vi "measure_j-v_keithley-2450.vi"(0 "User Name":string, 1 "Cell details cluster":T2={"Cell Position"=16, "Cell Label"="", "Pixel to measure"=0, "Area (cm^2)"=0.126, "Variable"="", "Variable value"="", "Scan settings in queue"=0, "Light or dark"="", "Measurement type"=""} {"Pixel to measure" items=["All", "1", "2", "3", "4", "5", "6", "7", "8"]}, 3 "Date array":string[](array[string]), 5 "Experiment Title":string, 12 "Scan settings":T1={"J-V scan"=TRUE, "Start voltage (V)"=0.0, "End voltage (V)"=0.0, "Step voltage (V)"=1.4, "Scan both directions"=TRUE, "Inverted device structure"=FALSE, "Settling delay (ms)"=10.0, "Measurement speed"=0, "Scan rate (V/s)"=0.0, "Stabilisation time (s)"=0.0, "Stabilisation mode"=0, "Stabilisation value (V or A) "=1.0, "Illumination"=0, "Stabilisation in the dark?"=FALSE, "Repeat light scans"=FALSE, "No. of repeat scans"=0.0, "Only repeat for best pixel"=1, "J-t scan"=FALSE, "J-t best pixel only"=7, "J-t start voltage (V)"=0.0, "J-t end voltage (V)"=1.4, "J-t step voltage (V)"=0.01, "Step time (s)"=0.7, "J-t scan both directions"=TRUE, "J-t inverted device structure"=FALSE, "J-t settling delay (ms)"=0.0, "J-t measurement speed"=0, "J-t illumination"=2, "Max. power stabilisation"=FALSE, "Max power best pixel only"=1, "Max. power point tracker"=FALSE, "Vmp from J-V scan"=FALSE, "Max P stab. Specific voltage"=FALSE, "Vmp (V)"=1.0, "Stabilisation time step (s)"=1.0, "Total stabilisation time (s)"=100.0} {"J-t settling delay (ms)" min=10.0; "J-t illumination" items=["Light only", "Dark only", "Light then dark", "Dark then light"]; "Measurement speed" items=["Fast", "Normal", "High accuracy"]; "Illumination" items=["Light only", "Dark only", "Light then dark", "Dark then light"]; "Only repeat for best pixel" items=["only for best pixel", "for best 2 pixels", "for best 3 pixels", "for best 4 pixels", "for best 5 pixels", "for best 6 pixels", "for best 7 pixels", "for all pixels"]; "No. of repeat scans" min=1.0 step=1.0; "Max power best pixel only" items=["only the best pixel", "the best 2 pixels", "the best 3 pixels", "the best 4 pixels", "the best 5 pixels", "the best 6 pixels", "the best 7 pixels", "all pixels"]; "J-t best pixel only" items=["only the best pixel", "the best 2 pixels", "the best 3 pixels", "the best 4 pixels", "the best 5 pixels", "the best 6 pixels", "the best 7 pixels", "all pixels"]; "J-t measurement speed" items=["Fast", "Normal", "High Accuracy"]; "Stabilisation mode" items=["V", "I"]; "Settling delay (ms)" min=10.0}, 13 "VISA resource name":refnum<visa-resource-name>="GPIB1::24::INSTR", 14 "Skip pixel?":bool) -> (4 "JV Curve":cluster{"Y":dbl[], "Y":dbl[]}[](graph), 6 "File path for master log":path, 15 "Log Table":string[][](table))   [LabVIEW 2016]
uses:
  <instrlib>/Keithley 2450/Keithley 2450.lvlib
  TypeDefs/scan_settings.ctl
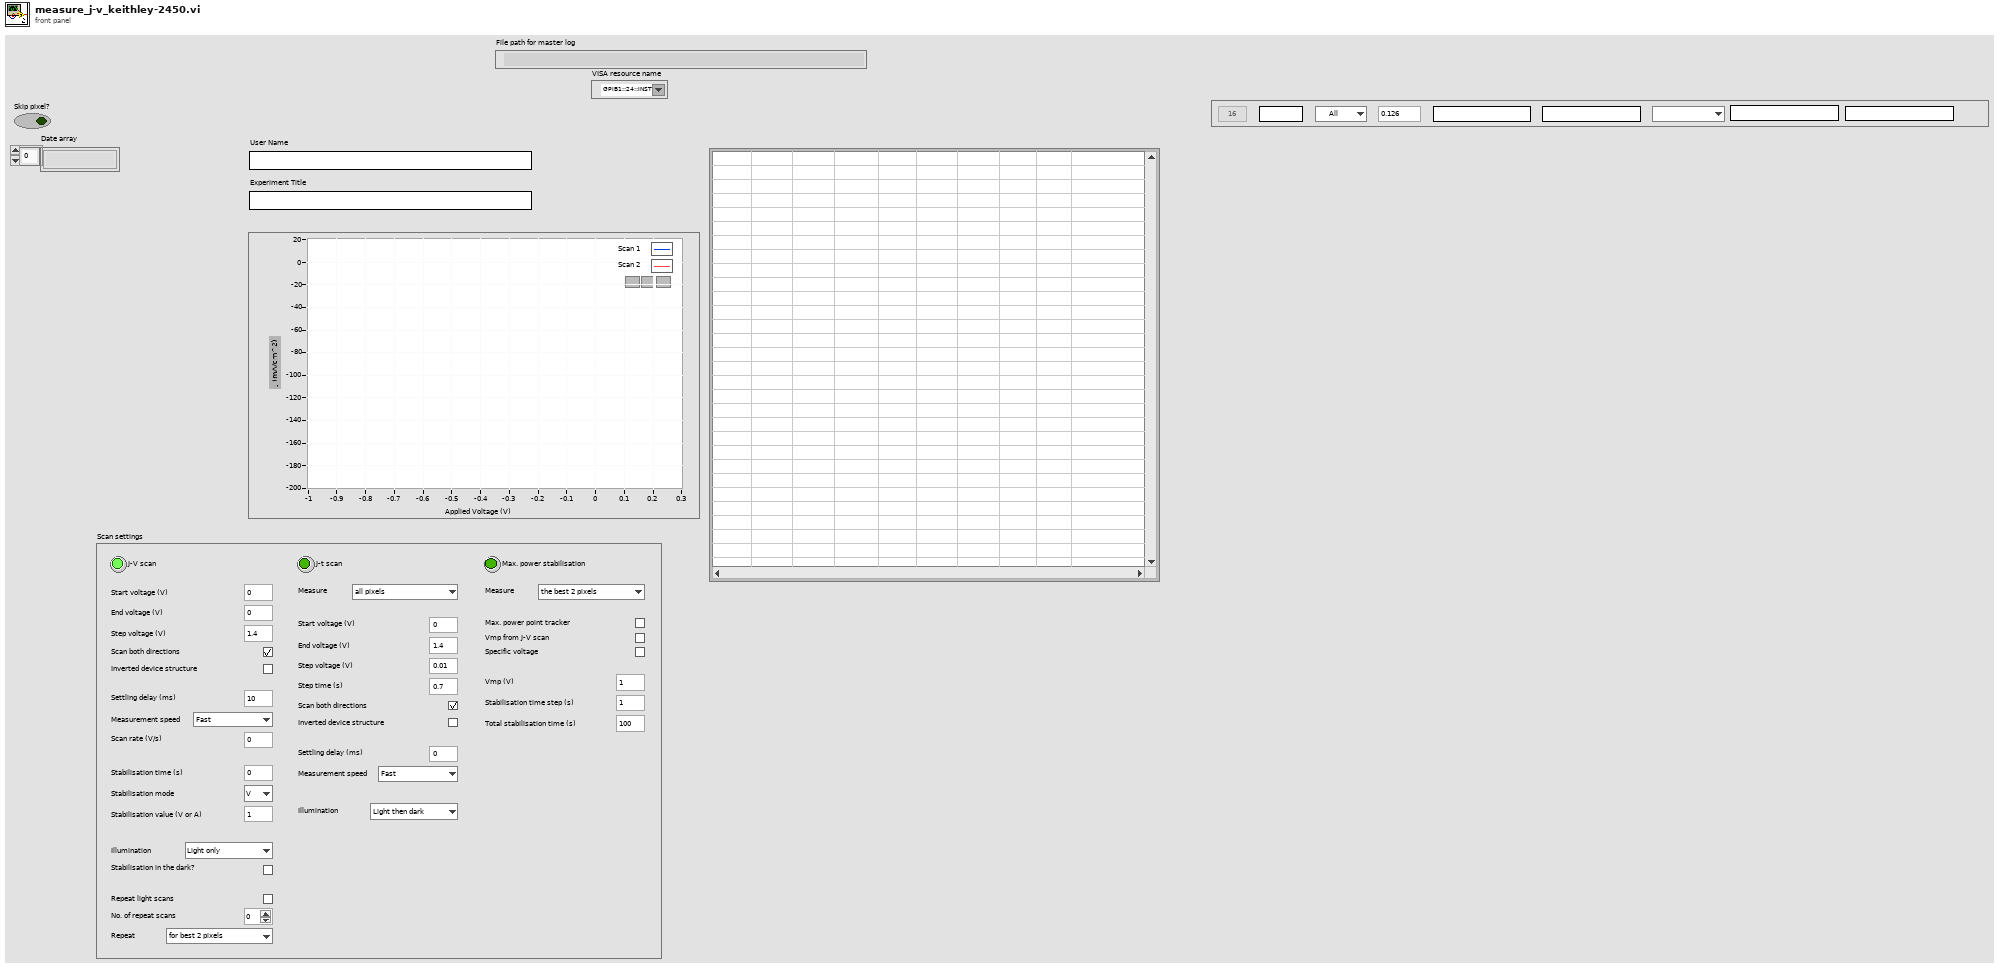
[diagram p1: front panel]
types:
  T1 = typedef "scan_settings.ctl" = cluster{"J-V scan":bool, "Start voltage (V)":dbl, "End voltage (V)":dbl, "Step voltage (V)":dbl, "Scan both directions":bool, "Inverted device structure":bool, "Settling delay (ms)":dbl, "Measurement speed":u8, "Scan rate (V/s)":dbl, "Stabilisation time (s)":dbl, "Stabilisation mode":u16, "Stabilisation value (V or A) ":dbl, "Illumination":u16, "Stabilisation in the dark?":bool, "Repeat light scans":bool, "No. of repeat scans":dbl, "Only repeat for best pixel":u16, "J-t scan":bool, "J-t best pixel only":u16, "J-t start voltage (V)":dbl, "J-t end voltage (V)":dbl, "J-t step voltage (V)":dbl, "Step time (s)":dbl, "J-t scan both directions":bool, "J-t inverted device structure":bool, "J-t settling delay (ms)":dbl, "J-t measurement speed":u16, "J-t illumination":u16, "Max. power stabilisation":bool, "Max power best pixel only":u16, "Max. power point tracker":bool, "Vmp from J-V scan":bool, "Max P stab. Specific voltage":bool, "Vmp (V)":dbl, "Stabilisation time step (s)":dbl, "Total stabilisation time (s)":dbl}
  T2 = cluster{"Cell Position":i32, "Cell Label":string, "Pixel to measure":u16, "Area (cm^2)":dbl, "Variable":string, "Variable value":string, "Scan settings in queue":u16, "Light or dark":string, "Measurement type":string}
  T3 = typedef "imagedata.ctl" = cluster{"image type":i32, "image depth":i32, "image":u8[], "mask":u8[], "colors":u32[], "Rectangle":cluster{"left":i16, "top":i16, "right":i16, "bottom":i16}}
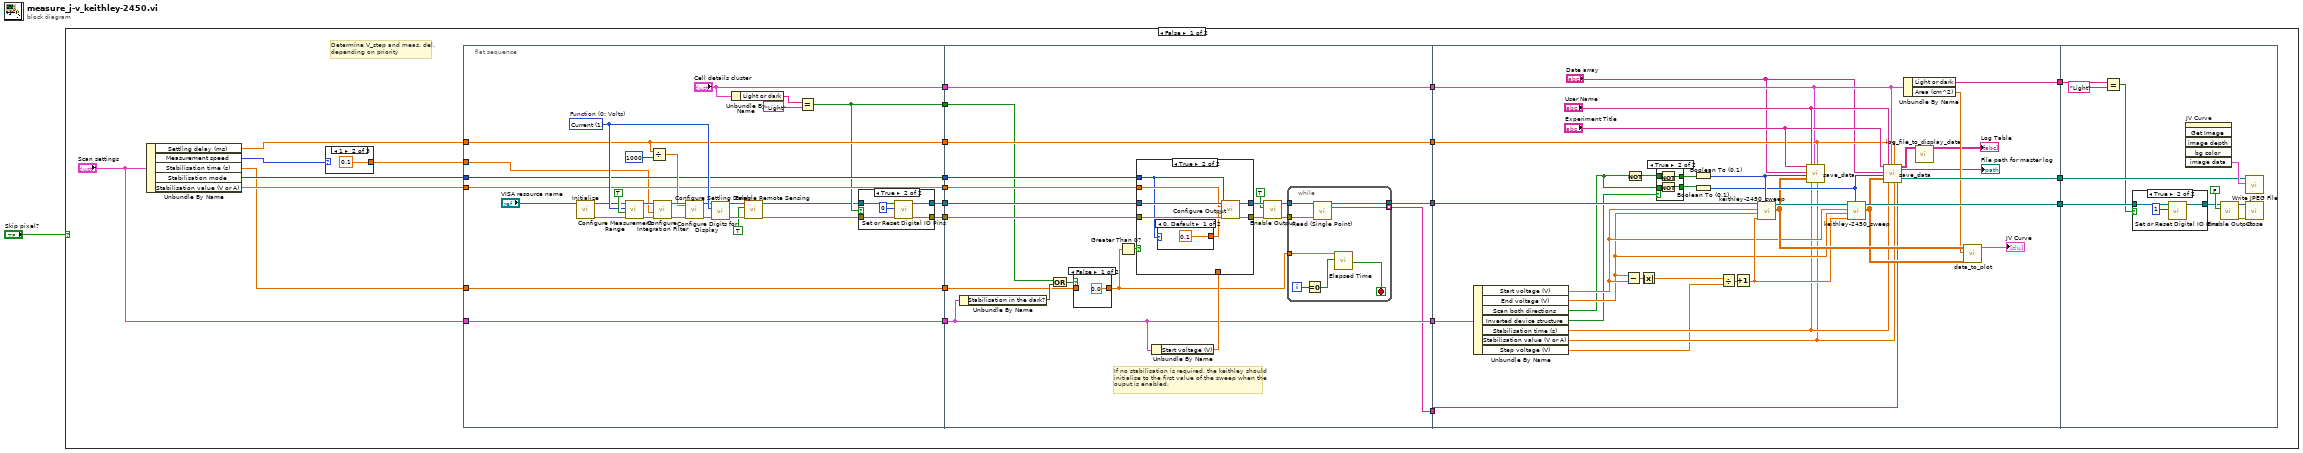
[diagram p0: block diagram]
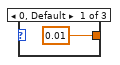
[diagram p2: hidden frame]
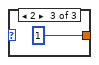
[diagram p3: hidden frame]
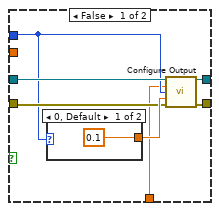
[diagram p6: hidden frame]
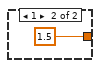
[diagram p7: hidden frame]
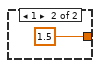
[diagram p8: hidden frame]
diagram:
  n1 = case shown="False" "Skip pixel?" {
    frame False {
      # "Determine V_step and meas. del.\ndepending on priority"
      n2 = Unbundle By Name("Scan settings") -> ("Settling delay (ms)"=w2:dbl, "Measurement speed"=w3:u8, "Stabilisation time (s)"=w5:dbl, "Stabilisation mode"=w7:u16, "Stabilisation value (V or A)"=w8:dbl)
      n3 = case shown="1" w3 {
        tunnel: [0.01 0.1 1] -> w4
        frame 0, Default {
        }
        frame 1 {
        }
        frame 2 {
        }
      }
      n4 = flat-sequence {
        tunnel: [w42] -> w25
        tunnel: [w35] -> w24
        tunnel: [w36] -> w23
        tunnel: w8 -> [w42]
        tunnel: [w41] -> w22
        tunnel: w7 -> [w41]
        tunnel: [w40] -> w21
        tunnel: w5 -> [w40]
        tunnel: w2 -> [w39]
        tunnel: [w39] -> w20
        tunnel: [w38] -> w19
        tunnel: "Scan settings" -> [w38]
        tunnel: ["Cell details cluster"] -> w18
        tunnel: [w32] -> w17
        tunnel: w4 -> [w31]
        tunnel: w25 -> [w78]
        tunnel: w24 -> [w83]
        tunnel: w23 -> [w84]
        tunnel: [w79] -> w16
        tunnel: [w66] -> w15
        tunnel: w22 -> [w75]
        tunnel: w21 -> [w67]
        tunnel: [w77] -> w14
        tunnel: w20 -> [w77]
        tunnel: [w72] -> w13
        tunnel: w19 -> [w72]
        tunnel: [w76] -> w12
        tunnel: w18 -> [w76]
        tunnel: w17 -> [w70]
        tunnel: [w142] -> w11
        tunnel: [w135] -> w10
        tunnel: w16 -> [w149]
        tunnel: w15 -> [w134]
        tunnel: w14 -> [w131]
        tunnel: w13 -> [w130]
        tunnel: w12 -> [w124]
        tunnel: [w123] -> w9
        tunnel: w11 -> [w160]
        tunnel: w10 -> [w161]
        tunnel: w9 -> [w156]
        frame #0 {
          w54 = u16 1 items=["Volts", "Current", "Resistance"]  # Function (0: Volts)
          n5 = call <instrlib>:"Initialize.vi"("VISA resource name"="VISA resource name") -> ("error out"=w44:errorcluster, "VISA resource name out"=w45:refnum<visa-resource-name>)  [unwired: 9 in]
          n6 = call <instrlib>:"Configure Measurement Range.vi"("error in (no error)"=w44, "Enable Auto Range (T:Enable)"=TRUE, "Function (0: Volts)"=w54, "VISA resource name"=w45) -> ("error out"=w47:errorcluster, "VISA resource name out"=w46:refnum<visa-resource-name>)  [unwired: 6 in]
          n7 = Divide(x=w39, y=1000) -> (x/y=w53:dbl)
          n8 = call <instrlib>:"Configure Integration Filter.vi"("error in (no error)"=w47, "Measurement Speed (1 PLC)"=w31, "VISA resource name"=w46) -> ("error out"=w56:errorcluster, "VISA resource name out"=w55:refnum<visa-resource-name>)  [unwired: 7 in]
          n9 = call <instrlib>:"Configure Settling Delay.vi"("Function (0: Volts)"=w53, "error in (no error)"=w56, "VISA resource name"=w55) -> ("error out"=w51:errorcluster, "VISA resource name out"=w50:refnum<visa-resource-name>)  [unwired: 7 in]
          n10 = call <instrlib>:"Configure Digits for Display.vi"("error in (no error)"=w51, "Function (0: Volts)"=w54, "VISA resource name"=w50) -> ("error out"=w49:errorcluster, "VISA resource name out"=w48:refnum<visa-resource-name>)  [unwired: 7 in]
          n11 = Unbundle By Name("Cell details cluster") -> ("Light or dark"=w34:string)
          n12 = call <instrlib>:"Enable Remote Sensing.vi"("error in (no error)"=w49, "Enable Remote Sensing (T: Enable)"=TRUE ("Enable Output (T: Enable)"), "VISA resource name"=w48) -> ("error out"=w29:errorcluster, "VISA resource name out"=w30:refnum<visa-resource-name>)  [unwired: 7 in]
          n13 = Equal?(x=w34, y="Light") -> (x = y?=w32:bool)
          n14 = case shown="True" w32 {
            tunnel: w30 -> [w60 w64]
            tunnel: w29 -> [w59 w63]
            tunnel: [w60 w62] -> w36
            tunnel: [w59 w61] -> w35
            frame False {
            }
            frame True {
              n15 = call <instrlib>:"Set or Reset Digital IO Pins.vi"("error in (no error)"=w63, "Digital IO Line (1)"=0, "VISA resource name"=w64) -> ("error out"=w61:errorcluster, "VISA resource name out"=w62:refnum<visa-resource-name>)  [unwired: 7 in]
            }
          }
        }
        frame #1 {
          # "If no stabilisation is required, the keithley should\ninitialise to the first value of the sweep when the\nouput is enabled."
          n16 = Unbundle By Name(w72) -> ("Stabilisation in the dark?"=w71:bool)
          n17 = Or(x=w70, y=w71) -> (x .or. y?=w69:bool)
          n18 = case shown="False" w69 {
            tunnel: [0.0 ("Stabilisation time (s)") w88] -> w68
            tunnel: w67 -> [_ w88]
            frame False {
            }
            frame True {
            }
          }
          n19 = Greater Than 0?(x=w68) -> (x > 0?=w74:bool)
          n20 = Unbundle By Name(w72) -> ("Start voltage (V)"=w73:dbl)
          n21 = case shown="True" w74 {
            tunnel: [w93 w104] -> w86
            tunnel: [w94 w103] -> w85
            tunnel: w84 -> [w91 w102]
            tunnel: w83 -> [w92 w101]
            tunnel: w78 -> [_ w100]
            tunnel: w75 -> [w90 w99]
            tunnel: w73 -> [w89 _]
            frame False {
              n22 = case shown="0, Default" w90 {
                tunnel: [0.1 1.5] -> w95
                frame 0, Default {
                }
                frame 1 {
                }
              }
              n23 = call <instrlib>:"Configure Output.vi"("VISA resource name"=w91, "Source Level (0)"=w89, "Source Mode  (0: Voltage)"=w90, "Source Limit Level (0.1)"=w95, "error in (no error)"=w92) -> ("VISA resource name out"=w94:refnum<visa-resource-name>, "error out"=w93:errorcluster)  [unwired: 9 in]
            }
            frame True {
              n24 = case shown="0, Default" w99 {
                tunnel: [0.1 1.5] -> w98
                frame 0, Default {
                }
                frame 1 {
                }
              }
              n25 = call <instrlib>:"Configure Output.vi"("VISA resource name"=w102, "Source Level (0)"=w100, "Source Mode  (0: Voltage)"=w99, "Source Limit Level (0.1)"=w98, "error in (no error)"=w101) -> ("VISA resource name out"=w103:refnum<visa-resource-name>, "error out"=w104:errorcluster)  [unwired: 9 in]
            }
          }
          n26 = call <instrlib>:"Enable Output.vi"("error in (no error)"=w86, "Enable Output (T: Enable)"=TRUE ("Output (Off)"), "VISA resource name"=w85) -> ("error out"=w80:errorcluster, "VISA resource name out"=w81:refnum<visa-resource-name>)  [unwired: 7 in]
          n27 = while {
            tunnel: w81 -> [w114]
            tunnel: w80 -> [w113]
            tunnel: [w112] -> w79
            tunnel: w68 -> [w108]
            tunnel: [w107] -> w66 mode=indexing
            i -> [w110]
            stop <- w111 stop-if-true
            n28 = Equal To 0?(x=w110) -> (x = 0?=w109:bool)
            n29 = call <instrlib>:"Read (Single Point).vi"("VISA resource name"=w114, "error in (no error)"=w113) -> ("VISA resource name out"=w112:refnum<visa-resource-name>, "Data out"=w107:string)  [unwired: 11 in, 1 out]
            n30 = call "Elapsed Time"("Time Target (s)"=w108, "Reset"=w109) -> ("Time has Elapsed"=w111:bool)  [unwired: 10 in, 7 out]
          }
        }
        frame #2 {
          n31 = Unbundle By Name(w130) -> ("Start voltage (V)"=w129:dbl, "End voltage (V)"=w128:dbl, "Scan both directions"=w118:bool, "Inverted device structure"=w127:bool, "Stabilisation time (s)"=w126:dbl, "Stabilisation value (V or A)"=w125:dbl, "Step voltage (V)"=w115:dbl)
          n32 = Subtract(x=w128, y=w129) -> (x-y=w147:dbl)
          n33 = Not(x=w118) -> (.not. x?=w119:bool)
          n34 = Absolute Value(x=w147) -> (abs(x)=w148:dbl)
          n35 = case shown="True" w127 {
            tunnel: [w151 w155] -> w137
            tunnel: [w150 w154] -> w136
            tunnel: w118 -> [w150 w153]
            tunnel: w119 -> [w151 w152]
            frame False {
            }
            frame True {
              n36 = Not(x=w152) -> (.not. x?=w155:bool)
              n37 = Not(x=w153) -> (.not. x?=w154:bool)
            }
          }
          n38 = Boolean To (0,1)(Boolean=w137) -> (0, 1=w145:i16)
          n39 = Boolean To (0,1)(Boolean=w136) -> (0, 1=w143:i16)
          n40 = Divide(x=w148, y=w115) -> (x/y=w139:dbl)
          n41 = Increment(x=w139) -> (x+1=w138:dbl)
          n42 = call "keithley-2450_sweep.vi"("Timeout (ms)"=w145, "Number of Points"=w138, "End voltage (V)"=w128, "Start voltage (V)"=w129, "VISA resource name out 2"=w149) -> ("Data Array"=w141:dbl[][], "VISA resource name out"=w144:refnum<visa-resource-name>)  [unwired: 2 in, 1 out]
          n43 = call "save_data.vi"("Experiment Indicator"="Experiment Title", "Date array"="Date array", "Scan direction"=w145, "Data Array"=w141, "Username"="User Name", "Stabilisation time (ms)"=w126, "Cell details cluster"=w124, "Measurement Delay (ms)"=w131, "Stabilisation level \n(A or V depending on mode)"=w125) -> ()  [unwired: 7 in, 4 out]
          n44 = call "keithley-2450_sweep.vi"("Scan direction"=w143, "Number of Points"=w138, "End voltage (V)"=w128, "Start voltage (V)"=w129, "VISA resource name out 2"=w144) -> ("Data Array"=w140:dbl[][], "VISA resource name out"=w142:refnum<visa-resource-name>)  [unwired: 2 in, 1 out]
          n45 = call "save_data.vi"("Experiment Indicator"="Experiment Title", "Date array"="Date array", "Scan direction"=w143, "Data Array"=w140, "Username"="User Name", "Stabilisation time (ms)"=w126, "Cell details cluster"=w124, "Measurement Delay (ms)"=w131, "Stabilisation level \n(A or V depending on mode)"=w125, "Stabilisation Data"=w134) -> ("Master Log"=w121:string[][], "File path for master log"=→"File path for master log":path, "File path for JV image"=w135:path)  [unwired: 6 in, 1 out]
          n46 = Unbundle By Name(w124) -> ("Light or dark"=w123:string, "Area (cm^2)"=w122:dbl)
          n47 = call "log_file_to_display_data.vi"("Master Log"=w121) -> ("Formatted table"=→"Log Table":string[][])  [unwired: 10 in]
          n48 = call "data_to_plot.vi"("Data Array 2"=w140, "Device Area (cm^2)"=w122, "Data Array"=w141) -> ("JV Curve"=→"JV Curve":cluster{"Y":dbl[], "Y":dbl[]}[])  [unwired: 8 in]
        }
        frame #3 {
          n49 = Equal?(x=w156, y="Light") -> (x = y?=w157:bool)
          n50 = case shown="True" w157 {
            tunnel: w160 -> [w166 w168]
            tunnel: [w166 w167] -> w159
            frame False {
            }
            frame True {
              n51 = call <instrlib>:"Set or Reset Digital IO Pins.vi"("Digital IO Line (1)"=1, "VISA resource name"=w168) -> ("VISA resource name out"=w167:refnum<visa-resource-name>)  [unwired: 8 in, 1 out]
            }
          }
          n52 = invoke on="JV Curve" class="XYGraph (strict)" method="Get Image"() -> ("image data"=w162:T3)  [unwired: 6 in, 5 out]
          n53 = call <instrlib>:"Enable Output.vi"("Enable Output (T: Enable)"=FALSE ("Output (Off)"), "VISA resource name"=w159) -> ("error out"=w164:errorcluster, "VISA resource name out"=w165:refnum<visa-resource-name>)  [unwired: 8 in]
          n54 = call <vilib>:"Write JPEG File.vi"("image data"=w162, "path to JPEG file"=w161) -> ()  [unwired: 8 in, 2 out]
          n55 = call <instrlib>:"Close.vi"("error in (no error)"=w164, "VISA resource name"=w165) -> ()  [unwired: 9 in, 1 out]
        }
      }
    }
    frame True {
    }
  }
